vi "2019-05-07_2.vi"() -> ()   [LabVIEW 2018]
panel:
  out "?":bool
  out "?":bool
  out "?":bool
  out "?":bool
  out "?":bool
  out "?":bool
  in  "빈 버튼 3":bool
  in  "빈 버튼 2":bool
  in  "빈 버튼":bool
  out "숫자형":dbl
  out "불리언":bool
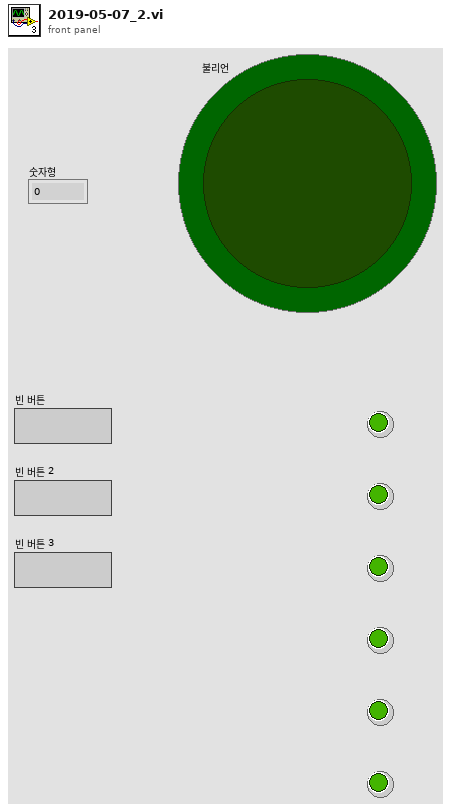
[diagram p1: front panel]
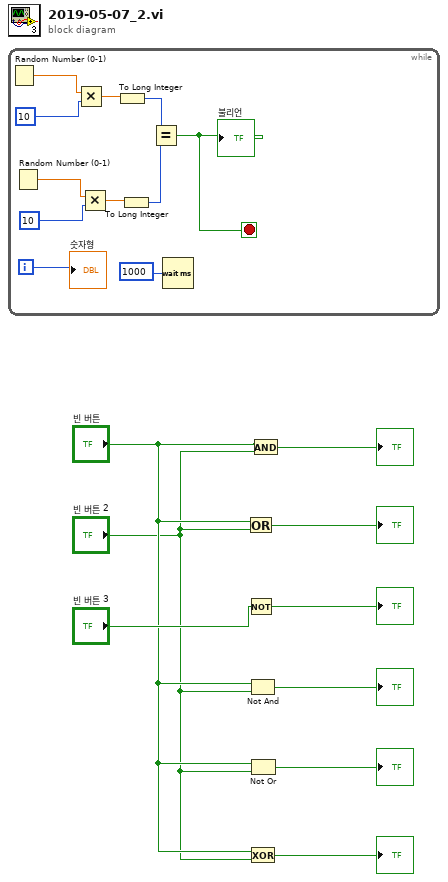
[diagram p0: block diagram]
diagram:
  n1 = while {
    i -> [w10]
    stop <- w12 stop-if-true
    n2 = Random Number (0-1)() -> (number: 0 to 1=w20:dbl)
    n3 = Random Number (0-1)() -> (number: 0 to 1=w16:dbl)
    n4 = Multiply(x=w20, y=10) -> (x*y=w18:dbl)
    n5 = Multiply(x=w16, y=10) -> (x*y=w14:dbl)
    n6 = To Long Integer(number=w18) -> (32bit integer=w17:i32)
    n7 = To Long Integer(number=w14) -> (32bit integer=w13:i32)
    n8 = Equal?(x=w17, y=w13) -> (x = y?=w12:bool)
    "불리언" <- w12
    n9 = Wait (ms)(milliseconds to wait=1000) -> ()  [unwired: 1 out]
    "숫자형" <- w10
  }
  n10 = Or(x="빈 버튼", y="빈 버튼 2") -> (x .or. y?=→"?":bool)
  n11 = Not(x="빈 버튼 3") -> (.not. x?=→"?":bool)
  n12 = Not And(1:"빈 버튼 2", 2:"빈 버튼") -> (0:→"?":bool)
  n13 = Not Or(1:"빈 버튼 2", 2:"빈 버튼") -> (0:→"?":bool)
  n14 = Exclusive Or(1:"빈 버튼 2", 2:"빈 버튼") -> (0:→"?":bool)
  n15 = And(x="빈 버튼", y="빈 버튼 2") -> (x .and. y?=→"?":bool)
